vi "Items Symbols to Flags.vi"(11 "Item Symbols":i32[](array[numeric])) -> (3 "Flags":bool[](array[boolean]))   [LabVIEW 2015, in "UIM.lvclass"]
uses:
  UIM.lvclass
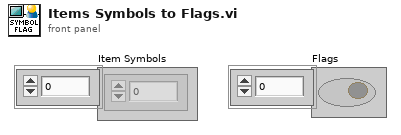
[diagram p1: front panel]
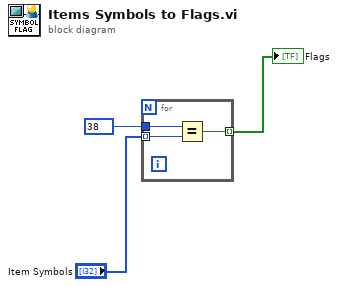
[diagram p0: block diagram]
diagram:
  n1 = for {
    tunnel: "Item Symbols" -> [w6] mode=indexing
    tunnel: 38 -> [w5]
    tunnel: [w4] -> w3 mode=indexing
    n2 = Equal?(x=w5, y=w6) -> (x = y?=w4:bool)
  }
  "Flags" <- w3
